vi "Get Color.vi"(11 "Orange Plugin in":refnum<class "Orange Plugin.lvclass">) -> (3 "Color Box":u32(colorbox))   [LabVIEW 2019, in "Orange Plugin.lvclass"]
uses:
  Orange Plugin.lvclass
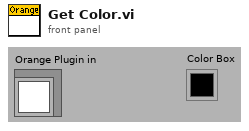
[diagram p1: front panel]
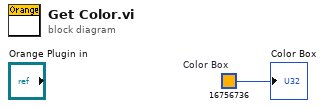
[diagram p0: block diagram]
diagram:
  w1 = u32 16756736  # Color Box
  "Color Box" <- w1
